vi "FindFirstTagC.vi"(8 "offset (0)":i32, 11 "XML String In":string) -> (0 "offset past match":i32, 1 "after tag":string, 2 "tag":string, 3 "before tag":string, 4 "case":enum16{"Start Tag", "Empty Element", "Content"}(ring), 5 "element name":string)   [LabVIEW 2017]
doc: "This VI finds the first XML tag (start tag or empty element tag) in the string and returns:\n\nbefore tag - portion of string prior to the tag\ntag - the contents of the tag including angle brackets (<,>)\nafter tag - portion of string found after the end of the tag\noffset past match - index in string of the first character of after substring\nelement name - the name (including namespace if applicable) of the element\ncase - whether a \"Start Tag\", \"Empty Element\", or \"Content\" (no tags) was found"
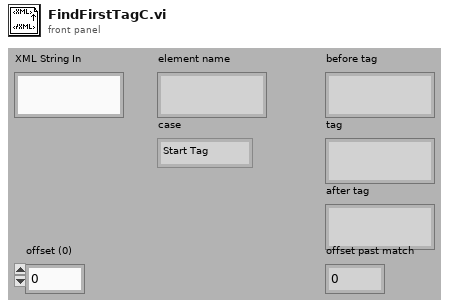
[diagram p1: front panel]
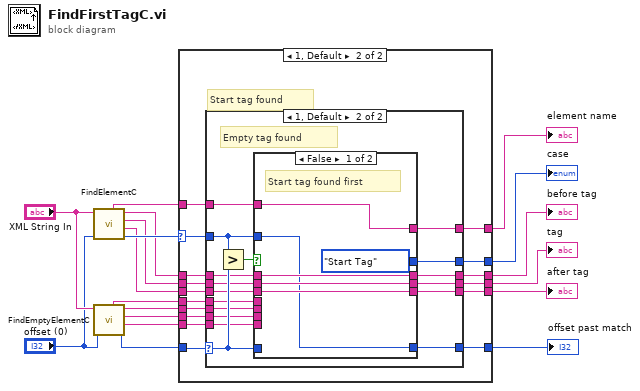
[diagram p0: block diagram]
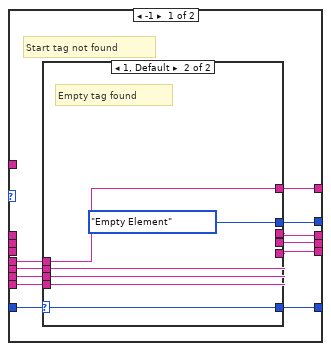
[diagram p2: hidden frame]
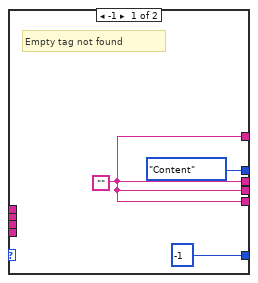
[diagram p3: hidden frame]
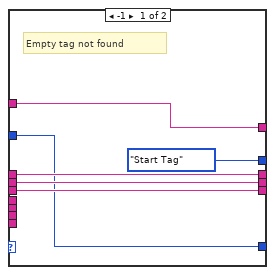
[diagram p4: hidden frame]
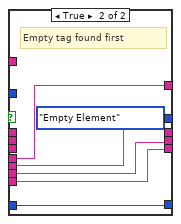
[diagram p5: hidden frame]
diagram:
  n1 = call "FindElementC.vi"("offset (0)"="offset (0)", "XML String In"="XML String In") -> ("offset past match"=w16:i32, "after  tag"=w13:string, "tag"=w14:string, "before tag"=w15:string, "element name"=w6:string)  [unwired: 5 in]
  n2 = call "FindEmptyElementC.vi"("offset (0)"="offset (0)", "XML String In"="XML String In") -> ("offset past match"=w11:i32, "after  tag"=w8:string, "tag"=w9:string, "before  tag"=w10:string, "element name"=w7:string)  [unwired: 5 in]
  n3 = case shown="1, Default" w16 {
    selector: w16 -> [_ w52]
    tunnel: [w28 w54] -> w1
    tunnel: w11 -> [w29 w53]
    tunnel: w10 -> [w27 w48]
    tunnel: w9 -> [w26 w47]
    tunnel: w8 -> [w25 w46]
    tunnel: w15 -> [_ w51]
    tunnel: w14 -> [_ w50]
    tunnel: w13 -> [_ w49]
    tunnel: [w24 w45] -> w18
    tunnel: [w23 w44] -> w5
    tunnel: [w22 w43] -> w17
    tunnel: w7 -> [w20 w42]
    tunnel: w6 -> [_ w41]
    tunnel: [w21 w40] -> w4
    tunnel: [w19 w39] -> w2
    frame -1 {
      # "Start tag not found"
      n4 = case shown="1, Default" w29 {
        selector: w29 -> [_ w34]
        tunnel: [enum16{"Start Tag", "Empty Element", "Content"}."Content" enum16{"Start Tag", "Empty Element", "Content"}."Empty Element"] -> w28
        tunnel: w27 -> [_ w38]
        tunnel: w26 -> [_ w37]
        tunnel: w25 -> [_ w36]
        tunnel: [w32 w38] -> w24
        tunnel: [w32 w37] -> w23
        tunnel: [w32 w36] -> w22
        tunnel: [w32 w35] -> w21
        tunnel: w20 -> [_ w35]
        tunnel: [-1 ("offset past match") w34] -> w19
        frame -1 {
          w32 = ""
          # "Empty tag not found"
        }
        frame 1, Default {
          # "Empty tag found"
        }
      }
    }
    frame 1, Default {
      # "Start tag found"
      n5 = case shown="1, Default" w53 {
        selector: w53 -> [_ w74]
        tunnel: [enum16{"Start Tag", "Empty Element", "Content"}."Start Tag" w77] -> w54
        tunnel: w52 -> [w56 w75]
        tunnel: w51 -> [w60 w73]
        tunnel: w50 -> [w59 w72]
        tunnel: w49 -> [w58 w71]
        tunnel: w48 -> [_ w70]
        tunnel: w47 -> [_ w69]
        tunnel: w46 -> [_ w68]
        tunnel: [w60 w67] -> w45
        tunnel: [w59 w66] -> w44
        tunnel: [w58 w65] -> w43
        tunnel: w42 -> [_ w64]
        tunnel: w41 -> [w57 w62]
        tunnel: [w57 w63] -> w40
        tunnel: [w56 w61] -> w39
        frame -1 {
          # "Empty tag not found"
        }
        frame 1, Default {
          # "Empty tag found"
          n6 = Greater?(x=w75, y=w74) -> (0:w76:bool)
          n7 = case shown="False" w76 {
            tunnel: [enum16{"Start Tag", "Empty Element", "Content"}."Start Tag" enum16{"Start Tag", "Empty Element", "Content"}."Empty Element"] -> w77
            tunnel: w75 -> [w79 _]
            tunnel: w74 -> [_ w85]
            tunnel: w73 -> [w83 _]
            tunnel: w72 -> [w82 _]
            tunnel: w71 -> [w81 _]
            tunnel: w70 -> [_ w89]
            tunnel: w69 -> [_ w88]
            tunnel: w68 -> [_ w87]
            tunnel: [w83 w89] -> w67
            tunnel: [w82 w88] -> w66
            tunnel: [w81 w87] -> w65
            tunnel: w64 -> [_ w86]
            tunnel: [w80 w86] -> w63
            tunnel: w62 -> [w80 _]
            tunnel: [w79 w85] -> w61
            frame False {
              # "Start tag found first"
            }
            frame True {
              # "Empty tag found first"
            }
          }
        }
      }
    }
  }
  "tag" <- w5
  "before tag" <- w18
  "after tag" <- w17
  "element name" <- w4
  "offset past match" <- w2
  "case" <- w1
